vi "Read Number of Test Methods.vi"(8 "error in (no error)":errorcluster, 11 "Test Finder In":refnum<class "Test Finder.lvclass">) -> (0 "error out":errorcluster, 2 "Number of Test Methods found":i32, 3 "Test Finder Out":refnum<class "Test Finder.lvclass">)   [LabVIEW 2020, in "Test Finder.lvclass"]
uses:
  Test Finder.lvclass
  Test Finder.lvclass/Test Finder.ctl
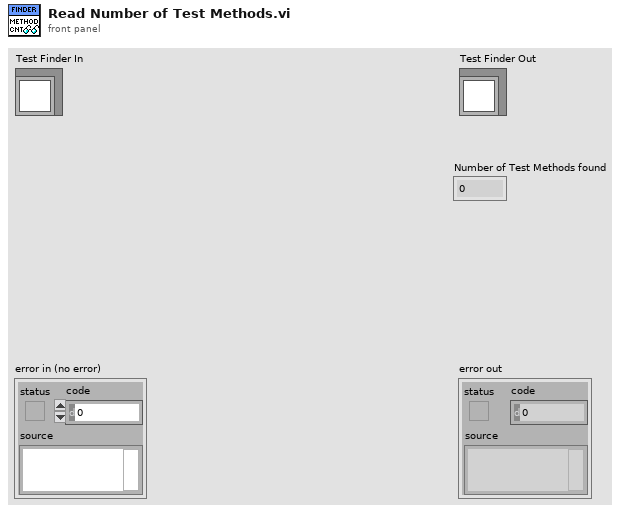
[diagram p1: front panel]
types:
  T1 = cluster{"Method Name":string, "Fully Qualified Name":string}[]
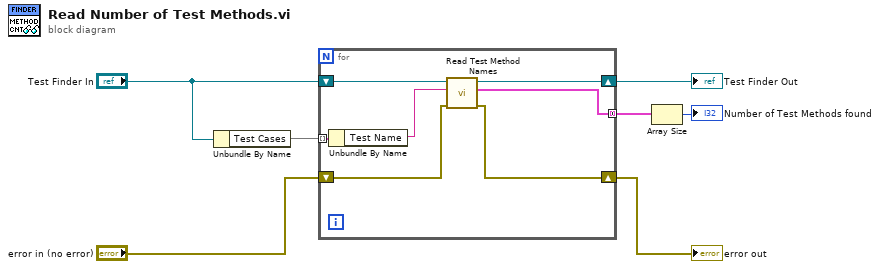
[diagram p0: block diagram]
diagram:
  n1 = Unbundle By Name("Test Finder In") -> ("Test Cases"=w7:map{string, path})
  n2 = for {
    tunnel: w7 -> [w12] mode=indexing
    shift-right: [w13] -> w5
    shift-left: "Test Finder In" -> [w14]
    shift-right: [w9] -> w3
    shift-left: "error in (no error)" -> [w10]
    tunnel: [w8] -> w2 mode=concatenating
    n3 = Unbundle By Name(w12) -> ("Test Name"=w11:string)
    n4 = call "Read Test Method Names.vi"("error in (no error)"=w10, "Test Case"=w11, "Test Case Finder In"=w14) -> ("error out"=w9:errorcluster, "Names"=w8:T1, "Test Case Finder Out"=w13:refnum<class "Test Finder.lvclass">)  [unwired: 6 in]
  }
  "error out" <- w3
  "Test Finder Out" <- w5
  n5 = Array Size(array=w2) -> (size(s)=→"Number of Test Methods found":i32)
